vi "Initialize CAN Frame.vi"(8 "error in":errorcluster, 10 "CAN Frame":T1={"Frame name"="frame1", "Identifier"=1, "Payload Length"=8, "Timing Type"=1, "Transmit Time"=0.0, "Extended Identifier?"=FALSE, "Comment"=""} {"Timing Type" items=["Cyclic Data", "Event Data", "Cyclic Remote", "Event Remote"]}, 11 "cluster in":refnum<k21>) -> (0 "error out":errorcluster, 2 "frame out":refnum<k21>, 3 "cluster out":refnum<k21>)   [LabVIEW 2015, in "Diagnostics Addon Shared.lvlib"]
uses:
  Diagnostics Addon Shared.lvlib
  Types/XNET.Frame.ctl
  <vilib>/xnet/xnet.llb/XNET Database Create (Frame).vi
  <resource>/objmgr/xnet.rc
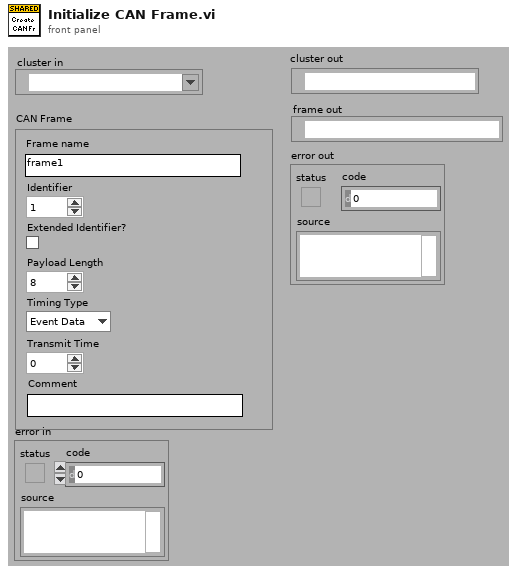
[diagram p1: front panel]
types:
  T1 = typedef "Diagnostics Addon Shared.lvlib/XNET.Frame.ctl" = cluster{"Frame name":string, "Identifier":u32, "Payload Length":u32, "Timing Type":u32, "Transmit Time":dbl, "Extended Identifier?":bool, "Comment":string}
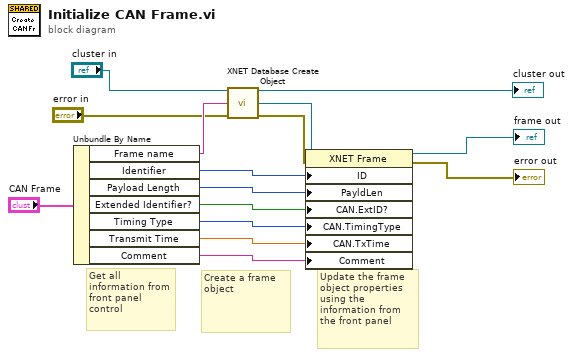
[diagram p0: block diagram]
diagram:
  # "Update the frame object properties using the information from the front panel"
  # "Create a frame object"
  # "Get all information from front panel control"
  n1 = Unbundle By Name("CAN Frame") -> ("Frame name"=w10:string, "Identifier"=w11:u32, "Payload Length"=w12:u32, "Extended Identifier?"=w13:bool, "Timing Type"=w14:u32, "Transmit Time"=w15:dbl, "Comment"=w2:string)
  n2 = call-poly <vilib>:"XNET Database Create Object.vi"("cluster in"="cluster in", "frame name"=w10, "error in (no error)"="error in") -> ("cluster out"=→"cluster out":refnum<k21>, "frame out"=w3:refnum<k21>, "error out"=w4:errorcluster)  [unwired: 10 in]
  n3 = property class="XNET Frame"(reference=w3, error in=w4, "ID"=w11, "PayldLen"=w12, "CAN.ExtID?"=w13, "CAN.TimingType"=w14, "CAN.TxTime"=w15, "Comment"=w2) -> (reference out=→"frame out":refnum<k21>, error out=→"error out":errorcluster)
